vi "GetTime.vi"(8 "error in (no error)":errorcluster, 11 "CarexMData in":refnum<class "ExpData.lvclass">) -> (0 "error out":errorcluster, 2 "Time":dbl[](array[numeric]), 3 "CarexMData out":refnum<class "ExpData.lvclass">)   [LabVIEW 2015, in "ExpData.lvclass"]
uses:
  ExpData.lvclass
panel:
  in  "Name (\"Time\")":string="Time"
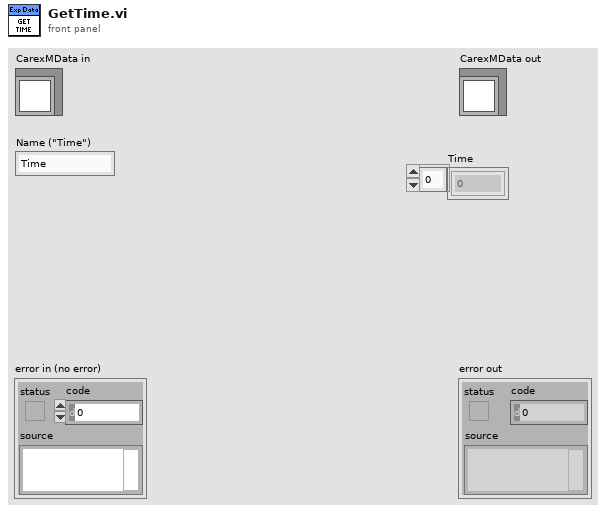
[diagram p1: front panel]
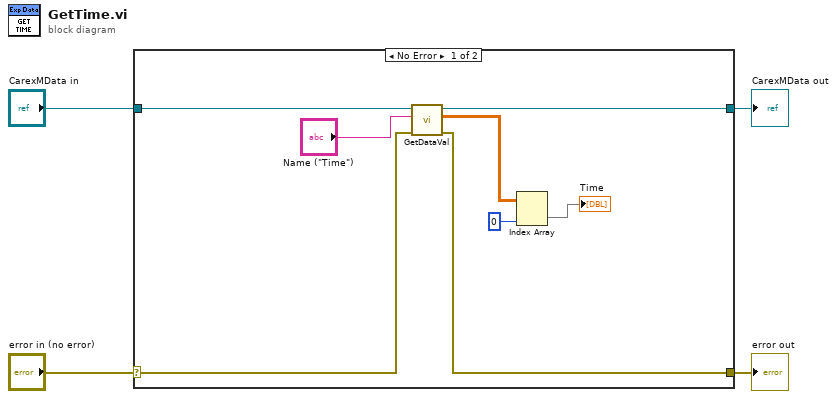
[diagram p0: block diagram]
diagram:
  n1 = case shown="No Error" "error in (no error)" {
    selector: "error in (no error)" -> [w10 w14]
    tunnel: [w9 w14] -> w3
    tunnel: [w11 w13] -> w1
    tunnel: "CarexMData in" -> [w12 w13]
    frame No Error {
      n2 = call "GetDataVal.vi"("error in (no error)"=w10, "Name"="Name (\"Time\")", "CarexMData in"=w12) -> ("error out"=w9:errorcluster, "Data"=w7:dbl[][], "CarexMData out"=w11:refnum<class "ExpData.lvclass">)  [unwired: 5 in, 1 out]
      n3 = Index Array(array=w7, index (col)=0 ("dimension size")) -> (element=→"Time":dbl[])  [unwired: 1 in]
    }
    frame Error {
    }
  }
  "error out" <- w3
  "CarexMData out" <- w1
